vi "FTW-CodeGen-Prototype.vi"(0 "ADAPT_Type and Defaults":cluster{"Element":variant}, 5 "REPLACE_JSON String":string, 7 "REPLACE_Element Path":string, 11 "REPLACE_error in":errorcluster) -> (4 "ADAPT_Values":cluster{"Element":variant}, 15 "REPLACE_error out":errorcluster)   [LabVIEW 2014, in "FTW-JSON-Fetch.xnode"]
uses:
  FTW-JSON-Fetch.xnode
  src/error/FTW-ERR-CallChain.vi
  src/string/FTW-STR-ReplaceWhitespace.vi
panel:
  # "Inputs"
  # "Outputs"
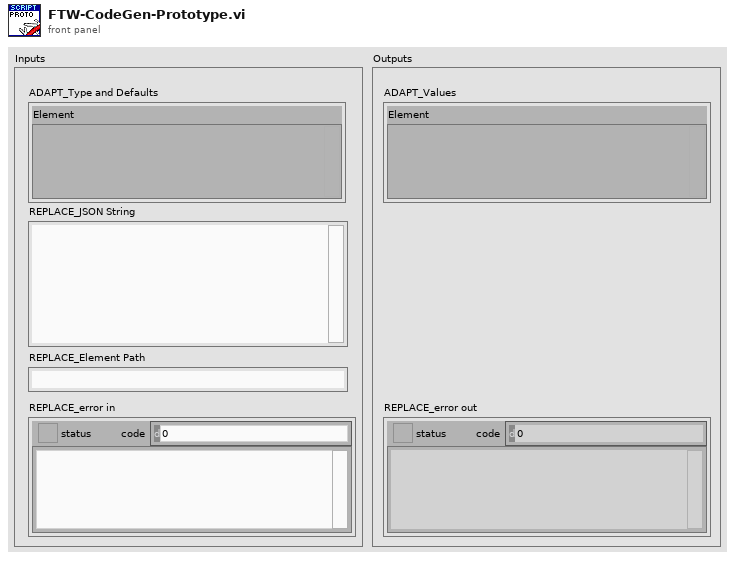
[diagram p1: front panel]
types:
  T1 = typedef "FTW-Reflection-Types.ctl" = enum16{"Unknown", "Void", "Array", "Cluster", "LVObject", "Boolean", "I8", "I16", "I32", "I64", "U8", "U16", "U32", "U64", "SGL", "DBL", "EXT", "CSG", "CDB", "CXT", "FXP", "EnumU8", "EnumU16", "EnumU32", "EnumU64", "SGLwithUnit", "DBLwithUnit", "EXTwithUnit", "CSGwithUnit", "CDBwithUnit", "CXTwithUnit", "String", "Path", "Picture", "Tag", "LVVariant", "Timestamp", "WaveformI8", "WaveformI16", "WaveformI32", "WaveformI64", "WaveformU8", "WaveformU16", "WaveformU32", "WaveformU64", "WaveformSGL", "WaveformDBL", "WaveformEXT", "WaveformCSG", "WaveformCDB", "WaveformCXT", "WaveformDigital", "WaveformUnknownType", "DigitalData", "DynamicData", "ExternalData", "FileByteStream", "TDMStream", "dotNET", "ActiveX", "VIServerReference", "VIReference", "ApplicationInstance", "Menu", "ConnectionDataSocket", "ConnectionVISA", "ConnectionBluetooth", "ConnectionIrDA", "ConnectionTCP", "ConnectionUDP", "ConnectionHTTPClient", "ConnectionFTP", "Occurrence", "Notifier", "Queue", "Rendezvous", "Semaphore", "RTFIFO", "EventPublisher", "EventRegistration", "EventCallback", "DataValueReference", "GenericClass", "GenericClassTag", "GenericClassDeepCopy", "GenericClassFlattened", "GenericClassTagFlattened", "GenericReferenceType", "WindowsRegistry", "OverloadedDatalogRef", "ReferenceUnknownType", "ByteArray", "ConPaneInterface"}
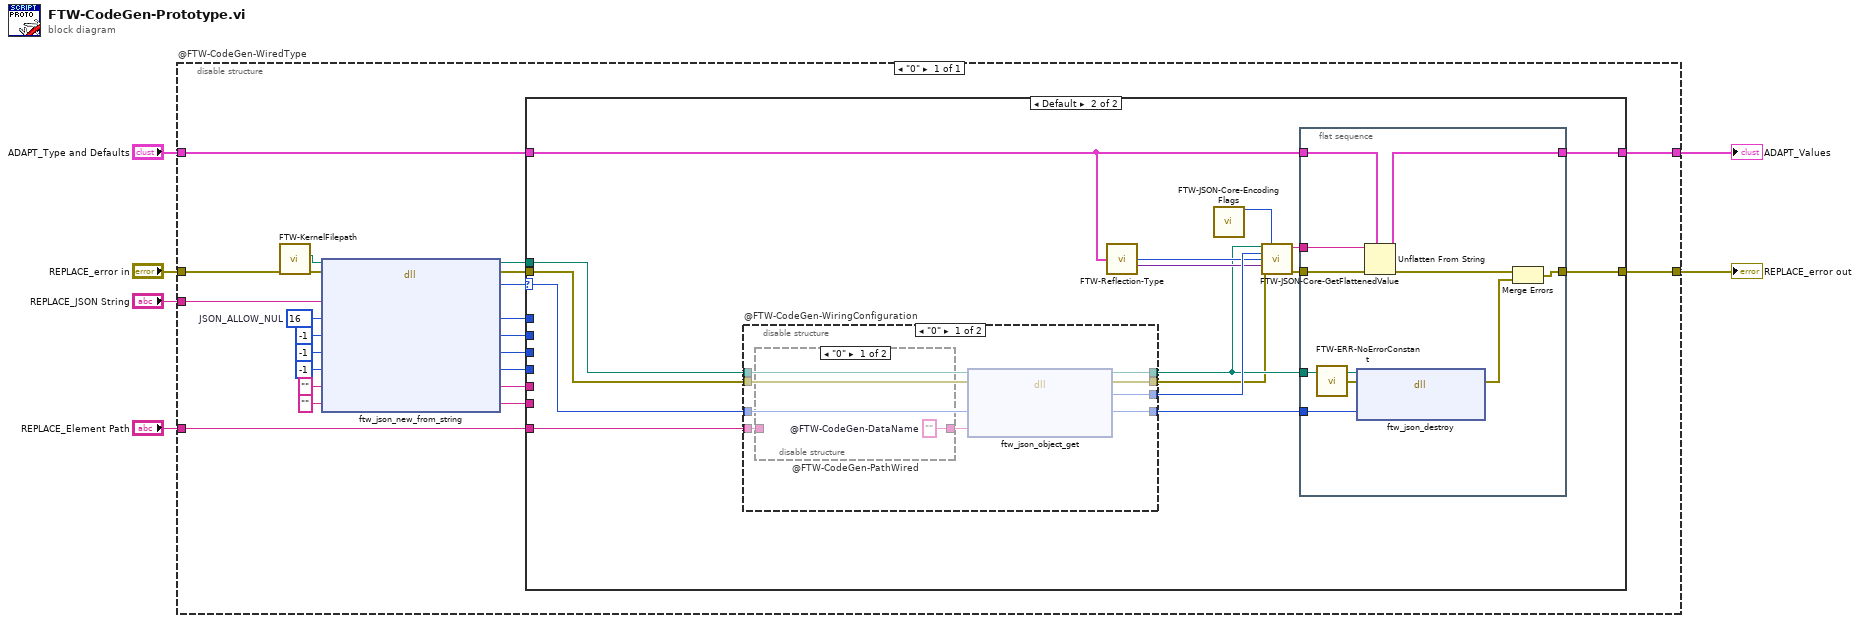
[diagram p0: block diagram]
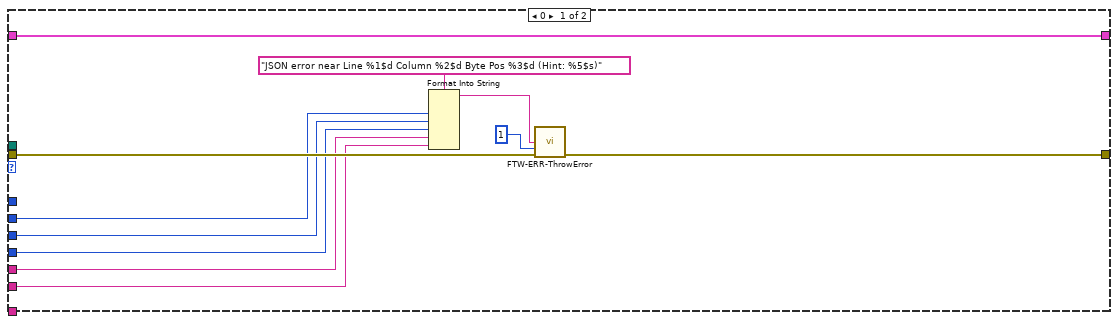
[diagram p2: hidden frame]
diagram:
  n1 = disable-structure "@FTW-CodeGen-WiredType" shown="\"0\"" {
    disable-tunnel: "ADAPT_Type and Defaults" -> [w29]
    disable-tunnel: [w28] -> w5
    disable-tunnel: "REPLACE_Element Path" -> [w27]
    disable-tunnel: "REPLACE_error in" -> [w18]
    disable-tunnel: "REPLACE_JSON String" -> [w17]
    disable-tunnel: [w8] -> w1
    frame condition #0 (active) {
      w19 = i64 16  # JSON_ALLOW_NUL
      n2 = call "FTW-KernelFilepath.vi"("error in"=w18) -> ("error out"=w21:errorcluster, "Library Filepath"=w20:path)  [unwired: 8 in, 1 out]
      n3 = dll-call lib="?" fn="ftw_json_new_from_string"(path in=w20, error in=w21, "JSON Buffer"=w17, "Flags"=w19, "Error Line Number"=i64 -1, "Error Column Number"=i64 -1, "Error Byte Position"=i64 -1, "Error Source"="", "Error Hint"="") -> (path out=w14:path, error out=w15:errorcluster, "JSON Object Pointer"=w16:i64, "Flags"=w7:i64, "Error Line Number"=w13:i64, "Error Column Number"=w12:i64, "Error Byte Position"=w11:i64, "Error Source"=w10:string, "Error Hint"=w9:string)  [unwired: 2 in]
      n4 = case shown="Default" w16 {
        selector: w16 -> [_ w46]
        tunnel: w29 -> [w31 w56]
        tunnel: [w31 w55] -> w28
        tunnel: w27 -> [_ w54]
        tunnel: w15 -> [w37 w47]
        tunnel: w14 -> [_ w45]
        tunnel: w13 -> [w36 _]
        tunnel: w12 -> [w35 _]
        tunnel: w11 -> [w34 _]
        tunnel: w10 -> [w33 _]
        tunnel: w9 -> [w32 _]
        tunnel: [w30 w44] -> w8
        tunnel: w7 -> [_ _]
        frame 0 {
          n5 = Format Into String(format string="JSON error near Line %1$d Column %2$d Byte Pos %3$d (Hint: %5$s)", w36, w35, w34, w33, w32) -> (resulting string=w39:string)  [unwired: 2 in, 1 out]
          n6 = call "FTW-ERR-ThrowError.vi"("Error Message"=w39, "Error Code"=1, "error in"=w37) -> ("error out"=w30:errorcluster)  [unwired: 12 in]
        }
        frame Default {
          n7 = disable-structure "@FTW-CodeGen-WiringConfiguration" shown="\"0\"" {
            disable-tunnel: w47 -> [w75 w80]
            disable-tunnel: [w74 w80] -> w41
            disable-tunnel: w46 -> [w73 w78]
            disable-tunnel: [w72 w78] -> w51
            disable-tunnel: w54 -> [w70 _]
            disable-tunnel: w45 -> [w69 w79]
            disable-tunnel: [w67 w79] -> w42
            disable-tunnel: [w68 w78] -> w43
            frame condition #0 {
              n8 = disable-structure "@FTW-CodeGen-PathWired" shown="\"0\"" {
                disable-tunnel: [w76 w77] -> w71
                disable-tunnel: w70 -> [_ w77]
                frame condition #0 (active) {
                  w76 = ""  # @FTW-CodeGen-DataName
                }
                frame condition #1 {
                }
              }
              n9 = dll-call lib="?" fn="ftw_json_object_get"(path in=w69, error in=w75, "JSON Object Pointer"=w73, "Element Key"=w71) -> (path out=w67:path, error out=w74:errorcluster, "JSON Element Pointer"=w72:i64, "JSON Object Pointer"=w68:i64)  [unwired: 2 in]
            }
            frame condition #1 (active) {
            }
          }
          n10 = call "FTW-Reflection-Type.vi"("Anything"=w56) -> ("LabVIEW Type"=w49:T1, "Variant Type and Value"=w50:variant)  [unwired: 12 in, 1 out]
          n11 = call "FTW-JSON-Core-EncodingFlags.vi"() -> ("Encoding Flags"=w48:i64)  [unwired: 14 in, 1 out]
          n12 = call "FTW-JSON-Core-GetFlattenedValue.vi"("Library Filepath"=w42, "JSON Element"=w51, "LabVIEW Type"=w49, "Element Default Value"=w50, "error in"=w41, "Encoding Flags"=w48) -> ("Flattened Value"=w53:string, "error out"=w52:errorcluster)  [unwired: 8 in]
          n13 = flat-sequence {
            tunnel: w56 -> [w66]
            tunnel: [w65] -> w55
            tunnel: w53 -> [w64]
            tunnel: w52 -> [w63]
            tunnel: [w58] -> w44
            tunnel: w42 -> [w62]
            tunnel: w43 -> [w61]
            frame #0 {
              n14 = call "FTW-ERR-NoErrorConstant.vi"() -> ("no error"=w57:errorcluster)
              n15 = dll-call lib="?" fn="ftw_json_destroy"(path in=w62, error in=w57, "JSON Object Pointer"=w61) -> (error out=w59:errorcluster)  [unwired: 3 in, 1 out]
              n16 = Unflatten From String(type=w66, binary string=w64, error in (no error)=w63) -> (value=w65:cluster{"Element":variant}, error out=w60:errorcluster)  [unwired: 2 in, 1 out]
              n17 = Merge Errors(w60, w59) -> (w58:errorcluster)
            }
          }
        }
      }
    }
  }
  "REPLACE_error out" <- w1
  "ADAPT_Values" <- w5
